vi "Cycling_No_DAQ_Tasks_All_3_PS.vi"() -> ()   [LabVIEW 2020]
uses:
  <instrlib>/NH Research Regenerative Test Series/Public/Configure/Output Safety.ctl
  Drivers-IT-M3400/IT-M3400.lvlib
  Drivers-Essentials/NH Research Regenerative Test Series.lvlib
panel:
  in  "Output Safety 3":T1
  in  "Output Safety 5":T1
  in  "Output Safety 4":T1
  in  "Battery Type 3":T2(ring)
  in  "Battery Type 5":T2(ring)
  in  "Mod # 3":enum16{"0", "1", "2"}(ring)
  in  "Mod # 5":enum16{"0", "1", "2"}(ring)
  in  "Mod # 4":enum16{"0", "1", "2"}(ring)
  in  "Number of Cycles 5":i32
  in  "Charge filepath 5":path
  in  "Discharge filepath 5":path
  in  "Batteryname 5":string
  in  "Starting Cycle 5":i32
  out "PS Visa Out 5":refnum<visa-resource-name>
  out "PS error out 5":errorcluster
  in  "Wait time 5":dbl
  in  "Discharge Current Setpoint 5":dbl format="%#.6g"
  in  "Charge Current Setpoint 5":dbl format="%#.6g"
  in  "PS type 5":enum16{"ITECH", "NHR"}(ring)
  in  "PS error in 5":errorcluster caption="PS error in     (no error)"
  in  "PS VISA in 5":refnum<visa-resource-name>
  in  "Number of Cycles 4":i32
  in  "Charge filepath 4":path
  in  "Discharge filepath 4":path
  in  "Batteryname 4":string
  in  "Starting Cycle 4":i32
  out "PS Visa Out 4":refnum<visa-resource-name>
  out "PS error out 4":errorcluster
  in  "Wait time 4":dbl
  in  "Discharge Current Setpoint 4":dbl format="%#.6g"
  in  "Charge Current Setpoint 4":dbl format="%#.6g"
  in  "Battery Type 4":T2(ring)
  in  "PS type 4":enum16{"ITECH", "NHR"}(ring)
  in  "PS error in 4":errorcluster caption="PS error in    (no error)"
  in  "PS VISA in 4":refnum<visa-resource-name>
  in  "Number of Cycles 3":i32
  in  "Charge filepath 3":path
  in  "Discharge filepath 3":path
  in  "Batteryname 3":string
  in  "Starting Cycle 3":i32
  out "PS Visa Out 3":refnum<visa-resource-name>
  out "PS error out 3":errorcluster
  in  "Wait time 3":dbl
  in  "Discharge Current Setpoint 3":dbl format="%#.6g"
  in  "Charge Current Setpoint 3":dbl format="%#.6g"
  in  "PS type 3":enum16{"ITECH", "NHR"}(ring)
  in  "PS error in 3":errorcluster caption="PS error in    (no error)"
  in  "PS VISA in 3":refnum<visa-resource-name>
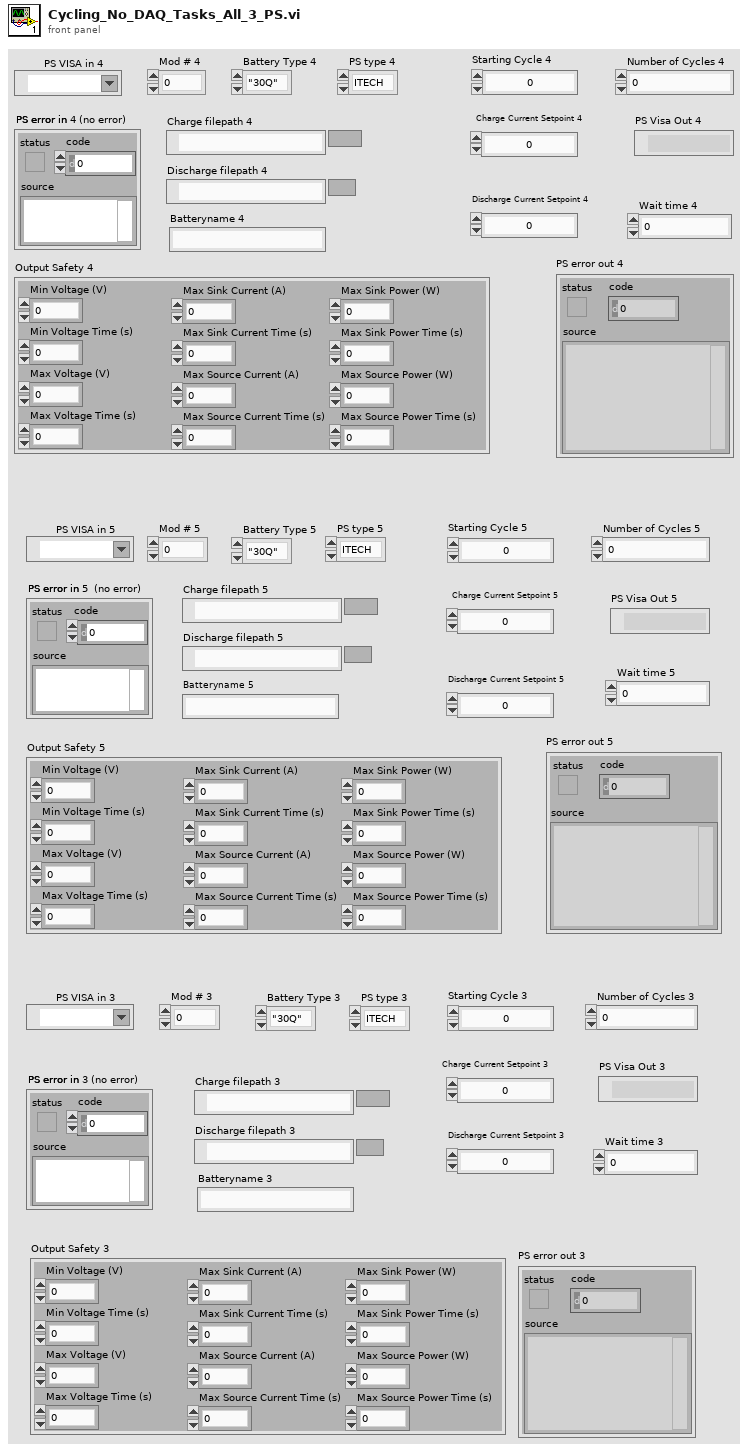
[diagram p1: front panel]
types:
  T1 = typedef "NH Research Regenerative Test Series.lvlib/Output Safety.ctl" = cluster{"Min Voltage (V)":dbl, "Min Voltage Time (s)":dbl, "Max Voltage (V)":dbl, "Max Voltage Time (s)":dbl, "Max Sink Current (A)":dbl, "Max Sink Current Time (s)":dbl, "Max Source Current (A)":dbl, "Max Source Current Time (s)":dbl, "Max Sink Power (W)":dbl, "Max Sink Power Time (s)":dbl, "Max Source Power (W)":dbl, "Max Source Power Time (s)":dbl}
  T2 = enum16{"\"30Q\"", "\"40T\"", "\"2P30Q\"", "\"3P30Q\"", "\"Nissan Leaf\"", ""}
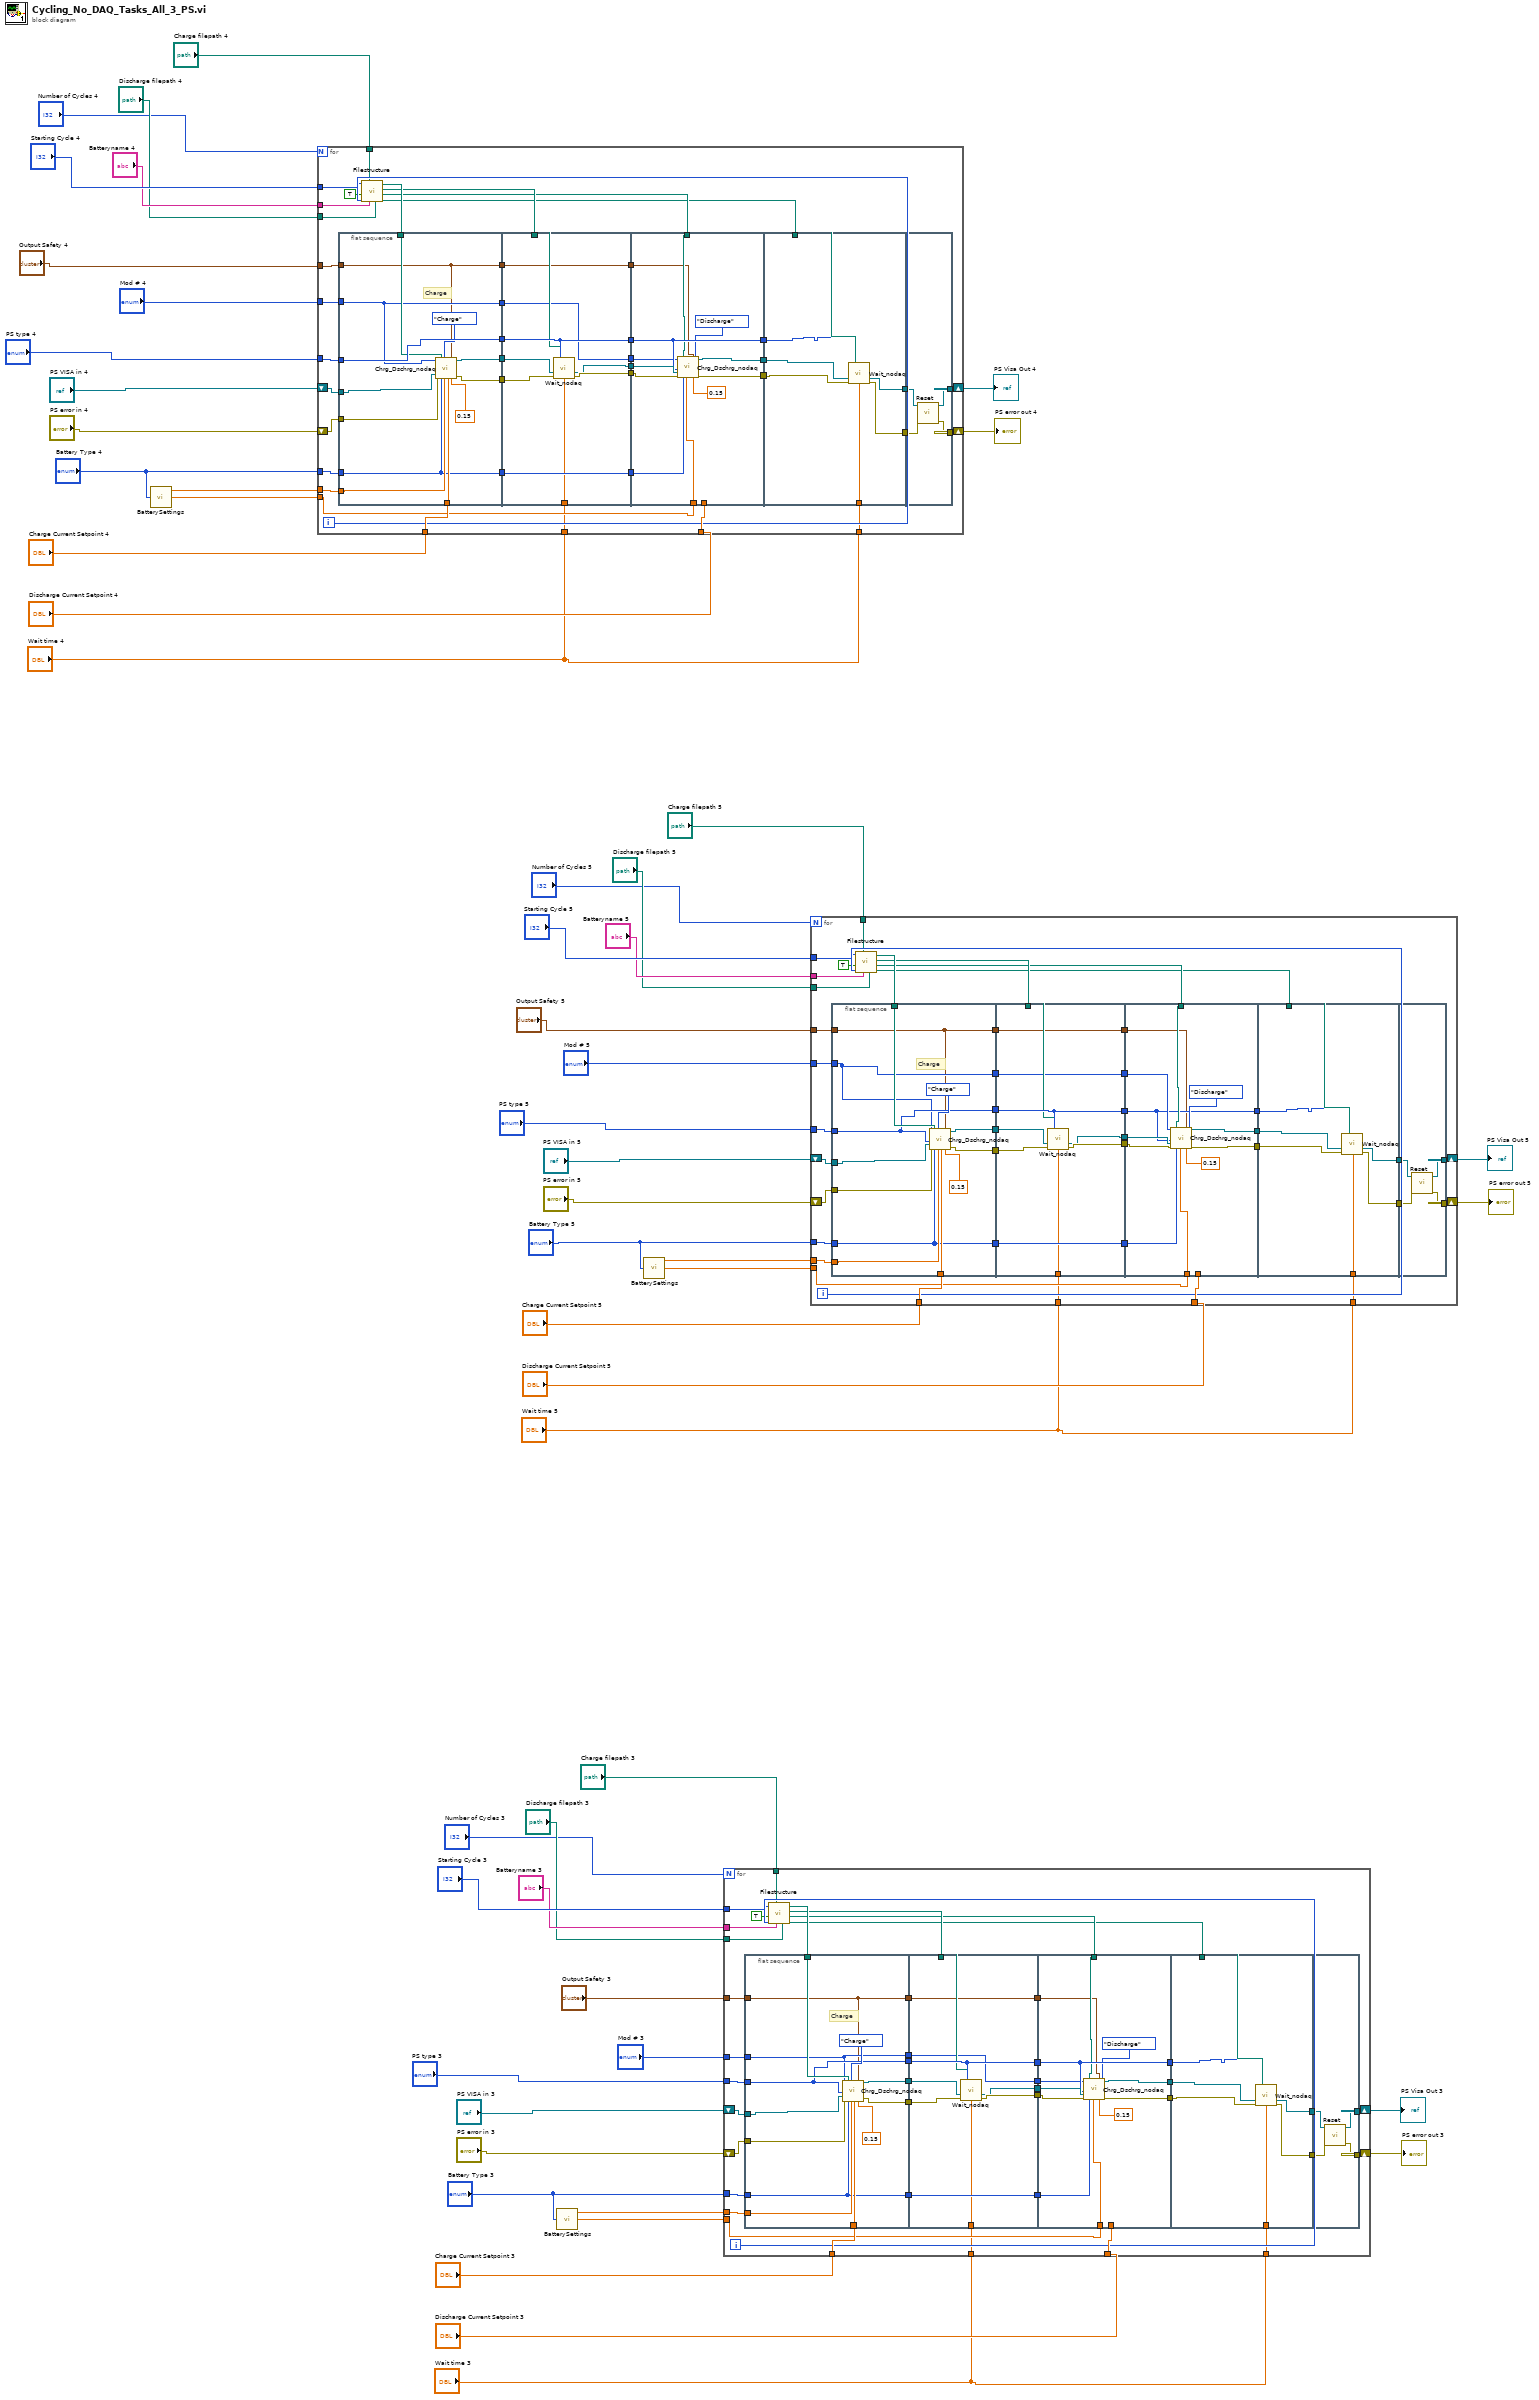
[diagram p0: block diagram]
diagram:
  n1 = call "BatterySettings.vi"("Battery Type"="Battery Type 4") -> ("Min Voltage (V)"=w33:dbl, "Max Voltage (V)"=w36:dbl)  [unwired: 2 in, 1 out]
  n2 = for {
    N: "Number of Cycles 4" -> [_]
    tunnel: "PS type 4" -> [w86]
    tunnel: w36 -> [w83]
    tunnel: "Battery Type 4" -> [w82]
    tunnel: "Charge Current Setpoint 4" -> [w81]
    tunnel: w33 -> [w80]
    tunnel: "Discharge Current Setpoint 4" -> [w79]
    shift-right: [w73] -> w30
    shift-left: "PS VISA in 4" -> [w85]
    shift-right: [w74] -> w31
    shift-left: "PS error in 4" -> [w84]
    tunnel: "Starting Cycle 4" -> [w71]
    tunnel: "Batteryname 4" -> [w69]
    tunnel: "Discharge filepath 4" -> [w68]
    tunnel: "Charge filepath 4" -> [w67]
    tunnel: "Wait time 4" -> [w62]
    tunnel: "Wait time 4" -> [w61]
    tunnel: "Mod # 4" -> [w60]
    tunnel: "Output Safety 4" -> [w57]
    i -> [w72]
    n3 = flat-sequence {
      tunnel: w86 -> [w108]
      tunnel: w85 -> [w99]
      tunnel: w84 -> [w100]
      tunnel: w82 -> [w97]
      tunnel: w83 -> [w101]
      tunnel: w81 -> [w102]
      tunnel: [w108] -> w95
      tunnel: [w97] -> w94
      tunnel: w78 -> [w107]
      tunnel: [w105] -> w64
      tunnel: [w104] -> w63
      tunnel: w60 -> [w98]
      tunnel: [w98] -> w59
      tunnel: w57 -> [w96]
      tunnel: [w96] -> w56
      tunnel: w95 -> [w117]
      tunnel: [w114] -> w93
      tunnel: [w115] -> w92
      tunnel: [w117] -> w91
      tunnel: w94 -> [w118]
      tunnel: [w118] -> w90
      tunnel: w77 -> [w116]
      tunnel: w64 -> [w113]
      tunnel: w63 -> [w112]
      tunnel: w61 -> [w111]
      tunnel: w59 -> [w110]
      tunnel: [w110] -> w58
      tunnel: w56 -> [w109]
      tunnel: [w109] -> w55
      tunnel: w93 -> [w126]
      tunnel: w92 -> [w127]
      tunnel: w91 -> [w125]
      tunnel: w90 -> [w129]
      tunnel: w80 -> [w128]
      tunnel: w79 -> [_]
      tunnel: w76 -> [w124]
      tunnel: [w121] -> w89
      tunnel: [w122] -> w88
      tunnel: [w125] -> w87
      tunnel: w58 -> [w120]
      tunnel: w55 -> [w119]
      tunnel: w75 -> [w136]
      tunnel: w89 -> [w137]
      tunnel: w88 -> [w134]
      tunnel: w87 -> [w132]
      tunnel: [w135] -> w66
      tunnel: [w133] -> w65
      tunnel: w62 -> [w131]
      tunnel: [w140] -> w73
      tunnel: [w138] -> w74
      tunnel: w66 -> [w139]
      tunnel: w65 -> [w141]
      frame #0 {
        # "Charge"
        n4 = call "Chrg_Dschrg_nodaq.vi"("Mod #"=w98, "PS VISA in"=w99, "PS error in"=w100, "CyclePath"=w107, "Battery Type"=w97, "Charge/discharge"=enum8{"Charge", "Discharge"}."Charge", "Charge/Discharge Voltage Setpoint"=w101, "Current Setpoint"=w102, "Output Safety"=w96, "Current Cutoff"=0.15) -> ("PS VISA out"=w105:refnum<visa-resource-name>, "PS error out"=w104:errorcluster)  [unwired: 8 in]
      }
      frame #1 {
        n5 = call "Wait_nodaq.vi"("PS type"=w117, "PS VISA in"=w113, "PS error in"=w112, "Wait Filepath"=w116, "Wait time"=w111) -> ("PS Visa Out"=w114:refnum<visa-resource-name>, "PS error out"=w115:errorcluster)  [unwired: 9 in]
      }
      frame #2 {
        n6 = call "Chrg_Dschrg_nodaq.vi"("Mod #"=w120, "PS type"=w125, "PS VISA in"=w126, "PS error in"=w127, "CyclePath"=w124, "Battery Type"=w129, "Charge/discharge"=enum8{"Charge", "Discharge"}."Discharge", "Charge/Discharge Voltage Setpoint"=w128, "Output Safety"=w119, "Current Cutoff"=0.15) -> ("PS VISA out"=w121:refnum<visa-resource-name>, "PS error out"=w122:errorcluster)  [unwired: 8 in]
      }
      frame #3 {
        n7 = call "Wait_nodaq.vi"("PS type"=w132, "PS VISA in"=w137, "PS error in"=w134, "Wait Filepath"=w136, "Wait time"=w131) -> ("PS Visa Out"=w133:refnum<visa-resource-name>, "PS error out"=w135:errorcluster)  [unwired: 9 in]
      }
      frame #4 {
        n8 = call <instrlib>:"Reset.vi"("error in"=w139, "VISA resource name"=w141) -> ("error out"=w138:errorcluster, "VISA resource name out"=w140:refnum<visa-resource-name>)  [unwired: 8 in]
      }
    }
    n9 = call "Filestructure.vi"("Discharge filepath"=w68, "Batteryname"=w69, "Charge filepath"=w67, "For loop i"=w72, "In for loop"=TRUE, "Starting Cycle"=w71) -> ("DischargeWaitPath"=w75:path, "DischargeCyclePath"=w76:path, "ChargeWaitPath"=w77:path, "ChargeCyclePath"=w78:path)  [unwired: 1 in, 1 out]
  }
  "PS error out 4" <- w31
  "PS Visa Out 4" <- w30
  n10 = call "BatterySettings.vi"("Battery Type"="Battery Type 3") -> ("Min Voltage (V)"=w49:dbl, "Max Voltage (V)"=w51:dbl)  [unwired: 2 in, 1 out]
  n11 = call "BatterySettings.vi"("Battery Type"="Battery Type 5") -> ("Min Voltage (V)"=w18:dbl, "Max Voltage (V)"=w20:dbl)  [unwired: 2 in, 1 out]
  n12 = for {
    N: "Number of Cycles 3" -> [_]
    tunnel: "PS type 3" -> [w173]
    tunnel: w51 -> [w170]
    tunnel: "Battery Type 3" -> [w169]
    tunnel: "Charge Current Setpoint 3" -> [w168]
    tunnel: w49 -> [w167]
    tunnel: "Discharge Current Setpoint 3" -> [w166]
    shift-right: [w160] -> w46
    shift-left: "PS VISA in 3" -> [w172]
    shift-right: [w161] -> w47
    shift-left: "PS error in 3" -> [w171]
    tunnel: "Starting Cycle 3" -> [w158]
    tunnel: "Batteryname 3" -> [w156]
    tunnel: "Discharge filepath 3" -> [w155]
    tunnel: "Charge filepath 3" -> [w154]
    tunnel: "Wait time 3" -> [w149]
    tunnel: "Wait time 3" -> [w148]
    tunnel: "Mod # 3" -> [w147]
    tunnel: "Output Safety 3" -> [w144]
    i -> [w159]
    n13 = flat-sequence {
      tunnel: w173 -> [w186]
      tunnel: w172 -> [w187]
      tunnel: w171 -> [w188]
      tunnel: w169 -> [w185]
      tunnel: w170 -> [w189]
      tunnel: w168 -> [w190]
      tunnel: [w186] -> w182
      tunnel: [w185] -> w181
      tunnel: w165 -> [w195]
      tunnel: [w193] -> w151
      tunnel: [w192] -> w150
      tunnel: w147 -> [w184]
      tunnel: [w184] -> w145
      tunnel: w144 -> [w183]
      tunnel: [w183] -> w143
      tunnel: w182 -> [w204]
      tunnel: [w201] -> w180
      tunnel: [w202] -> w179
      tunnel: [w204] -> w178
      tunnel: w181 -> [w205]
      tunnel: [w205] -> w177
      tunnel: w164 -> [w203]
      tunnel: w151 -> [w200]
      tunnel: w150 -> [w199]
      tunnel: w148 -> [w198]
      tunnel: [w197] -> w146
      tunnel: w145 -> [w197]
      tunnel: w143 -> [w196]
      tunnel: [w196] -> w142
      tunnel: w180 -> [w213]
      tunnel: w179 -> [w214]
      tunnel: w178 -> [w212]
      tunnel: w177 -> [w216]
      tunnel: w167 -> [w215]
      tunnel: w166 -> [_]
      tunnel: w163 -> [w211]
      tunnel: [w208] -> w176
      tunnel: [w209] -> w175
      tunnel: [w212] -> w174
      tunnel: w146 -> [w207]
      tunnel: w142 -> [w206]
      tunnel: w162 -> [w223]
      tunnel: w176 -> [w224]
      tunnel: w175 -> [w221]
      tunnel: w174 -> [w219]
      tunnel: [w222] -> w153
      tunnel: [w220] -> w152
      tunnel: w149 -> [w218]
      tunnel: [w227] -> w160
      tunnel: [w225] -> w161
      tunnel: w153 -> [w226]
      tunnel: w152 -> [w228]
      frame #0 {
        # "Charge"
        n14 = call "Chrg_Dschrg_nodaq.vi"("Mod #"=w184, "PS type"=w186, "PS VISA in"=w187, "PS error in"=w188, "CyclePath"=w195, "Battery Type"=w185, "Charge/discharge"=enum8{"Charge", "Discharge"}."Charge", "Charge/Discharge Voltage Setpoint"=w189, "Current Setpoint"=w190, "Output Safety"=w183, "Current Cutoff"=0.15) -> ("PS VISA out"=w193:refnum<visa-resource-name>, "PS error out"=w192:errorcluster)  [unwired: 7 in]
      }
      frame #1 {
        n15 = call "Wait_nodaq.vi"("PS type"=w204, "PS VISA in"=w200, "PS error in"=w199, "Wait Filepath"=w203, "Wait time"=w198) -> ("PS Visa Out"=w201:refnum<visa-resource-name>, "PS error out"=w202:errorcluster)  [unwired: 9 in]
      }
      frame #2 {
        n16 = call "Chrg_Dschrg_nodaq.vi"("Mod #"=w207, "PS type"=w212, "PS VISA in"=w213, "PS error in"=w214, "CyclePath"=w211, "Battery Type"=w216, "Charge/discharge"=enum8{"Charge", "Discharge"}."Discharge", "Charge/Discharge Voltage Setpoint"=w215, "Output Safety"=w206, "Current Cutoff"=0.15) -> ("PS VISA out"=w208:refnum<visa-resource-name>, "PS error out"=w209:errorcluster)  [unwired: 8 in]
      }
      frame #3 {
        n17 = call "Wait_nodaq.vi"("PS type"=w219, "PS VISA in"=w224, "PS error in"=w221, "Wait Filepath"=w223, "Wait time"=w218) -> ("PS Visa Out"=w220:refnum<visa-resource-name>, "PS error out"=w222:errorcluster)  [unwired: 9 in]
      }
      frame #4 {
        n18 = call <instrlib>:"Reset.vi"("error in"=w226, "VISA resource name"=w228) -> ("error out"=w225:errorcluster, "VISA resource name out"=w227:refnum<visa-resource-name>)  [unwired: 8 in]
      }
    }
    n19 = call "Filestructure.vi"("Discharge filepath"=w155, "Batteryname"=w156, "Charge filepath"=w154, "For loop i"=w159, "In for loop"=TRUE, "Starting Cycle"=w158) -> ("DischargeWaitPath"=w162:path, "DischargeCyclePath"=w163:path, "ChargeWaitPath"=w164:path, "ChargeCyclePath"=w165:path)  [unwired: 1 in, 1 out]
  }
  "PS error out 3" <- w47
  "PS Visa Out 3" <- w46
  n20 = for {
    N: "Number of Cycles 5" -> [_]
    tunnel: "PS type 5" -> [w260]
    tunnel: w20 -> [w257]
    tunnel: "Battery Type 5" -> [w256]
    tunnel: "Charge Current Setpoint 5" -> [w255]
    tunnel: w18 -> [w254]
    tunnel: "Discharge Current Setpoint 5" -> [w253]
    shift-right: [w247] -> w15
    shift-left: "PS VISA in 5" -> [w259]
    shift-right: [w248] -> w16
    shift-left: "PS error in 5" -> [w258]
    tunnel: "Starting Cycle 5" -> [w245]
    tunnel: "Batteryname 5" -> [w243]
    tunnel: "Discharge filepath 5" -> [w242]
    tunnel: "Charge filepath 5" -> [w241]
    tunnel: "Wait time 5" -> [w236]
    tunnel: "Wait time 5" -> [w235]
    tunnel: "Mod # 5" -> [w234]
    tunnel: "Output Safety 5" -> [w231]
    i -> [w246]
    n21 = flat-sequence {
      tunnel: w260 -> [w272]
      tunnel: w259 -> [w274]
      tunnel: w258 -> [w275]
      tunnel: w256 -> [w273]
      tunnel: w257 -> [w276]
      tunnel: w255 -> [w277]
      tunnel: [w272] -> w269
      tunnel: [w273] -> w268
      tunnel: w252 -> [w282]
      tunnel: [w280] -> w238
      tunnel: [w279] -> w237
      tunnel: w234 -> [w271]
      tunnel: [w271] -> w232
      tunnel: w231 -> [w270]
      tunnel: [w270] -> w230
      tunnel: w269 -> [w291]
      tunnel: [w288] -> w267
      tunnel: [w289] -> w266
      tunnel: [w291] -> w265
      tunnel: w268 -> [w292]
      tunnel: [w292] -> w264
      tunnel: w251 -> [w290]
      tunnel: w238 -> [w287]
      tunnel: w237 -> [w286]
      tunnel: w235 -> [w285]
      tunnel: [w284] -> w233
      tunnel: w232 -> [w284]
      tunnel: w230 -> [w283]
      tunnel: [w283] -> w229
      tunnel: w267 -> [w300]
      tunnel: w266 -> [w301]
      tunnel: w265 -> [w294]
      tunnel: w264 -> [w303]
      tunnel: w254 -> [w302]
      tunnel: w253 -> [_]
      tunnel: w250 -> [w299]
      tunnel: [w296] -> w263
      tunnel: [w297] -> w262
      tunnel: [w294] -> w261
      tunnel: w233 -> [w295]
      tunnel: w229 -> [w293]
      tunnel: w249 -> [w310]
      tunnel: w263 -> [w311]
      tunnel: w262 -> [w308]
      tunnel: w261 -> [w306]
      tunnel: [w309] -> w240
      tunnel: [w307] -> w239
      tunnel: w236 -> [w305]
      tunnel: [w314] -> w247
      tunnel: [w312] -> w248
      tunnel: w240 -> [w313]
      tunnel: w239 -> [w315]
      frame #0 {
        # "Charge"
        n22 = call "Chrg_Dschrg_nodaq.vi"("Mod #"=w271, "PS type"=w272, "PS VISA in"=w274, "PS error in"=w275, "CyclePath"=w282, "Battery Type"=w273, "Charge/discharge"=enum8{"Charge", "Discharge"}."Charge", "Charge/Discharge Voltage Setpoint"=w276, "Current Setpoint"=w277, "Output Safety"=w270, "Current Cutoff"=0.15) -> ("PS VISA out"=w280:refnum<visa-resource-name>, "PS error out"=w279:errorcluster)  [unwired: 7 in]
      }
      frame #1 {
        n23 = call "Wait_nodaq.vi"("PS type"=w291, "PS VISA in"=w287, "PS error in"=w286, "Wait Filepath"=w290, "Wait time"=w285) -> ("PS Visa Out"=w288:refnum<visa-resource-name>, "PS error out"=w289:errorcluster)  [unwired: 9 in]
      }
      frame #2 {
        n24 = call "Chrg_Dschrg_nodaq.vi"("Mod #"=w295, "PS type"=w294, "PS VISA in"=w300, "PS error in"=w301, "CyclePath"=w299, "Battery Type"=w303, "Charge/discharge"=enum8{"Charge", "Discharge"}."Discharge", "Charge/Discharge Voltage Setpoint"=w302, "Output Safety"=w293, "Current Cutoff"=0.15) -> ("PS VISA out"=w296:refnum<visa-resource-name>, "PS error out"=w297:errorcluster)  [unwired: 8 in]
      }
      frame #3 {
        n25 = call "Wait_nodaq.vi"("PS type"=w306, "PS VISA in"=w311, "PS error in"=w308, "Wait Filepath"=w310, "Wait time"=w305) -> ("PS Visa Out"=w307:refnum<visa-resource-name>, "PS error out"=w309:errorcluster)  [unwired: 9 in]
      }
      frame #4 {
        n26 = call <instrlib>:"Reset.vi"("error in"=w313, "VISA resource name"=w315) -> ("error out"=w312:errorcluster, "VISA resource name out"=w314:refnum<visa-resource-name>)  [unwired: 8 in]
      }
    }
    n27 = call "Filestructure.vi"("Discharge filepath"=w242, "Batteryname"=w243, "Charge filepath"=w241, "For loop i"=w246, "In for loop"=TRUE, "Starting Cycle"=w245) -> ("DischargeWaitPath"=w249:path, "DischargeCyclePath"=w250:path, "ChargeWaitPath"=w251:path, "ChargeCyclePath"=w252:path)  [unwired: 1 in, 1 out]
  }
  "PS error out 5" <- w16
  "PS Visa Out 5" <- w15
